vi "EvaluateOpStateExit.vi"(8 "error in (no error)":errorcluster, 9 "data":T2, 10 "config in":T1, 11 "Qbus in":refnum<class "Qbus.lvclass">) -> (0 "error out":errorcluster, 2 "config out":T1, 3 "Qbus out":refnum<class "Qbus.lvclass">)   [LabVIEW 2017, in "McsaDataEventCreator.lvlib"]
uses:
  <vilib>/addons/InsightCM/Devices/Shared/Mcsa/McsaDataEventCreator/McsaDataEventCreator.lvlib
  <vilib>/addons/InsightCM/Devices/Shared/Common/DataFlow/controls/Data.ctl
  <vilib>/addons/InsightCM/Utilities/DataAccessors/controls/wfmSGL_DVR.ctl
  <vilib>/addons/PointValueMap/controls/PointMap.ctl
  <vilib>/addons/InsightCM/Devices/Shared/Common/DataFlow/controls/Type.ctl
  <vilib>/addons/Qbus/Qbus.lvclass
  <vilib>/addons/InsightCM/Devices/Shared/Mcsa/McsaDataEventCreator/controls/config.ctl
  <vilib>/addons/InsightCM/Devices/Shared/Mcsa/McsaDataEventCreator/controls/AcqParams.ctl
  <vilib>/addons/InsightCM/Devices/Shared/Common/DataAccumulator/controls/AccumulationSettings.ctl
  <vilib>/addons/InsightCM/Devices/Shared/Common/DataAccumulator/controls/accumulationType.ctl
  <vilib>/addons/InsightCM/Devices/Shared/Common/DVRBuffer/controls/BufferLocation.ctl
  <vilib>/addons/InsightCM/Devices/Shared/Mcsa/McsaDataEventCreator/controls/DataEventConfig.ctl
  <vilib>/addons/InsightCM/Devices/Shared/Common/DataEventCreator/controls/Reason.ctl
  <vilib>/addons/PointValueMap/subVIs/Point_Read_string.vi
  <vilib>/addons/PointValueMap/PointValueMap.lvlib
  <vilib>/addons/InsightCM/Devices/Shared/Common/DataEventCreator/DataEventCreator.lvlib
  <vilib>/addons/InsightCM/Devices/Shared/Common/DVRBuffer/DVRBuffer.lvlib
  <vilib>/addons/InsightCM/Devices/Shared/Common/DataAccumulator/DataAccumulator.lvlib
  <vilib>/addons/InsightCM/Devices/Shared/Common/DataFlow/DataFlow.lvlib
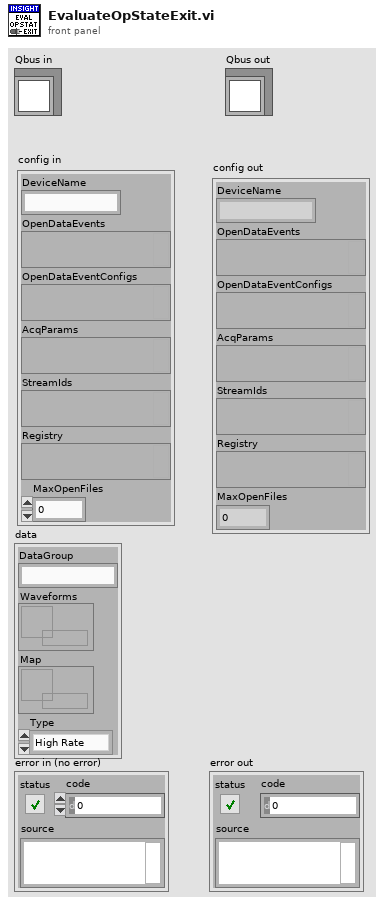
[diagram p1: front panel]
types:
  T1 = typedef "McsaDataEventCreator.lvlib/config.ctl" = cluster{"DeviceName":string, "OpenDataEvents":variant, "OpenDataEventConfigs":variant, "AcqParams":variant, "StreamIds":variant, "Registry":variant, "MaxOpenFiles":i32}
  T2 = typedef "DataFlow.lvlib/Data.ctl" = cluster{"DataGroup":string, "Waveforms":T3, "Map":T4, "Type":T5}
  T3 = typedef "wfmSGL_DVR.ctl" = refnum<data-value>
  T4 = typedef "PointValueMap.lvlib/PointMap.ctl" = refnum<data-value>
  T5 = typedef "DataFlow.lvlib/Type.ctl" = enum16{"High Rate", "Low Rate", "Burst Mode"}
  T6 = typedef "McsaDataEventCreator.lvlib/AcqParams.ctl" = cluster{"Stream":bool, "PreTrigger":i32, "CollectOnEnter":bool, "Enter PreTrigger":i32, "Enter Length":dbl, "CollectOnExit":bool, "ContinuousData":bool, "Accumulation Settings":T7}
  T7 = typedef "DataAccumulator.lvlib/AccumulationSettings.ctl" = cluster{"Type":T8, "Length":dbl, "Max Time (sec)":dbl, "Start Block":T9, "Acquired (sec)":dbl, "Acquired (pulses)":i32, "Initial Pulse Offset":dbl, "Stop Block":T9, "LastBlockAdded":u32}
  T8 = typedef "DataAccumulator.lvlib/accumulationType.ctl" = enum16{"none", "seconds", "revolutions"}
  T9 = typedef "DVRBuffer.lvlib/BufferLocation.ctl" = cluster{"Block":u32, "Index":i32}
  T10 = typedef "DataEventCreator.lvlib/Reason.ctl" = enum16{"Periodic Event", "Delta EU Event", "Trend Event", "Alarm Event", "User Event", "Enter Operating State", "Exit Operating State", "Multiple Events", "Other"}
  T11 = typedef "McsaDataEventCreator.lvlib/DataEventConfig.ctl" = cluster{"AcqParams":T6, "OpState":string, "ExitOpState":bool, "Reason":string, "StreamId":string, "Map":T4, "DataSetIds":variant, "IncludeWaveforms":bool, "TrendPointsOnly":bool}
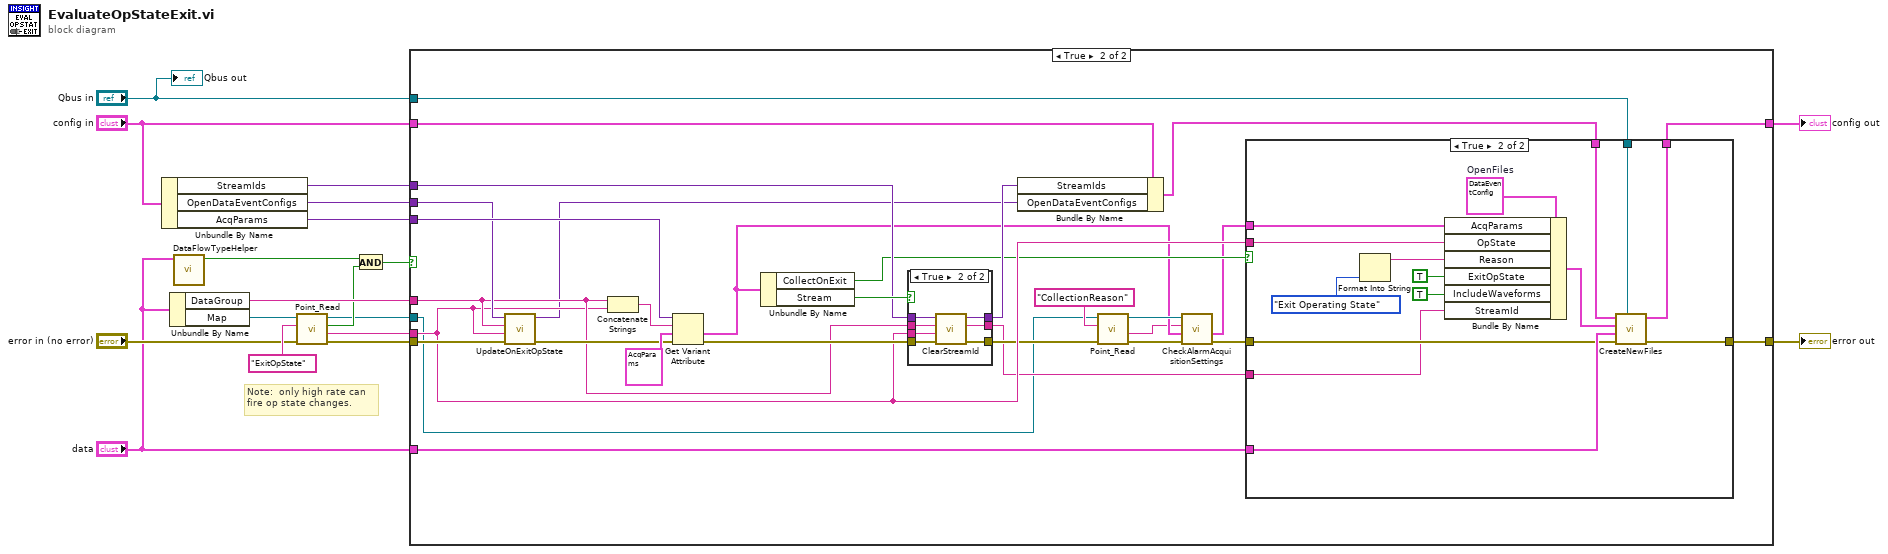
[diagram p0: block diagram]
diagram:
  # "Note:  only high rate can\nfire op state changes."
  n1 = Unbundle By Name("config in") -> ("StreamIds"=w12:variant, "OpenDataEventConfigs"=w8:variant, "AcqParams"=w7:variant)
  n2 = Unbundle By Name("data") -> ("DataGroup"=w13:string, "Map"=w18:T4)
  n3 = call <vilib>:"DataFlowTypeHelper.vi"("data"="data") -> ("high rate"=w1:bool)  [unwired: 8 in, 2 out]
  n4 = call-poly <vilib>:"Point_Read.vi"("Error In"="error in (no error)", "Tag"="ExitOpState", "Map"=w18) -> ("Error Out"=w15:errorcluster, "Value"=w14:string, "Found?"=w5:bool, "Map Out"=w3:T4)  [unwired: 3 in, 2 out]
  n5 = And(x=w1, y=w5) -> (x .and. y?=w4:bool)
  n6 = case shown="True" w4 {
    tunnel: w15 -> [w19 w37]
    tunnel: w14 -> [_ w33]
    tunnel: w13 -> [_ w34]
    tunnel: w7 -> [_ w49]
    tunnel: w12 -> [_ w45]
    tunnel: "config in" -> [w20 w44]
    tunnel: [w20 w43] -> w10
    tunnel: "data" -> [_ w42]
    tunnel: "Qbus in" -> [_ w41]
    tunnel: [w19 w40] -> w9
    tunnel: w8 -> [_ w35]
    tunnel: w3 -> [_ w25]
    frame False {
    }
    frame True {
      n7 = call <vilib>:"UpdateOnExitOpState.vi"("error in (no error)"=w37, "operating state"=w33, "data group"=w34, "open data event configs in"=w35) -> ("error out"=w36:errorcluster, "open data event configs out"=w32:variant)  [unwired: 6 in]
      n8 = Concatenate Strings(w34, w33) -> (w50:string)
      n9 = Get Variant Attribute(Variant=w49, name=w50, default value (empty Variant)=T6 {"Stream"=FALSE, "PreTrigger"=0, "CollectOnEnter"=FALSE, "Enter PreTrigger"=0, "Enter Length"=0.0, "CollectOnExit"=FALSE, "ContinuousData"=FALSE, "Accumulation Settings"={"Type"=enum."none", "Length"=0.0, "Max Time (sec)"=0.0, "Start Block"={"Block"=0, "Index"=0}, "Acquired (sec)"=0.0, "Acquired (pulses)"=0, "Initial Pulse Offset"=0.0, "Stop Block"={"Block"=0, "Index"=0}, "LastBlockAdded"=0}} ("AcqParams"), error in=w36) -> (value=w22:T6, error out=w46:errorcluster)  [unwired: 2 out]
      n10 = Unbundle By Name(w22) -> ("CollectOnExit"=w31:bool, "Stream"=w47:bool)
      n11 = case shown="True" w47 {
        tunnel: w46 -> [w68 w76]
        tunnel: w45 -> [w69 w75]
        tunnel: w34 -> [_ w74]
        tunnel: w33 -> [_ w73]
        tunnel: [w69 w72] -> w39
        tunnel: [_ w71] -> w27
        tunnel: [w68 w70] -> w29
        frame False {
        }
        frame True {
          n12 = call <vilib>:"ClearStreamId.vi"("error in (no error)"=w76, "operating state"=w73, "data group"=w74, "OpStateCorrIds in"=w75) -> ("error out"=w70:errorcluster, "operating state corrId"=w71:string, "OpStateCorrIds out"=w72:variant)  [unwired: 5 in]
        }
      }
      n13 = Bundle By Name(cluster=w44, "StreamIds"=w39, "OpenDataEventConfigs"=w32) -> (w38:T1)
      n14 = call-poly <vilib>:"Point_Read.vi"("Error In"=w29, "Tag"="CollectionReason", "Map"=w25) -> ("Error Out"=w24:errorcluster, "Value"=w21:string, "Map Out"=w26:T4)  [unwired: 3 in, 3 out]
      n15 = call <vilib>:"CheckAlarmAcquisitionSettings.vi"("error in (no error)"=w24, "acq config in"=w22, "collection reason"=w21, "map"=w26) -> ("error out"=w28:errorcluster, "acq config out"=w23:T6)  [unwired: 6 in]
      n16 = case shown="True" w31 {
        tunnel: w23 -> [_ w67]
        tunnel: [w52 w66] -> w43
        tunnel: w42 -> [_ w65]
        tunnel: w41 -> [_ w64]
        tunnel: [w51 w63] -> w40
        tunnel: w28 -> [w51 w62]
        tunnel: w38 -> [w52 w61]
        tunnel: w33 -> [_ w60]
        tunnel: w27 -> [_ w54]
        frame False {
        }
        frame True {
          w59 = T11 {"AcqParams"={"Stream"=FALSE, "PreTrigger"=0, "CollectOnEnter"=FALSE, "Enter PreTrigger"=0, "Enter Length"=0.0, "CollectOnExit"=FALSE, "ContinuousData"=FALSE, "Accumulation Settings"={"Type"=enum."none", "Length"=0.0, "Max Time (sec)"=0.0, "Start Block"={"Block"=0, "Index"=0}, "Acquired (sec)"=0.0, "Acquired (pulses)"=0, "Initial Pulse Offset"=0.0, "Stop Block"={"Block"=0, "Index"=0}, "LastBlockAdded"=0}}, "OpState"="", "ExitOpState"=FALSE, "Reason"="", "StreamId"="", "Map"=refnum, "DataSetIds"=variant, "IncludeWaveforms"=FALSE, "TrendPointsOnly"=FALSE}  # OpenFiles
          n17 = Format Into String(Reason."Exit Operating State" ("Reason")) -> (resulting string=w55:string)  [unwired: 3 in, 1 out]
          n18 = Bundle By Name(cluster=w59, "AcqParams"=w67, "OpState"=w60, "Reason"=w55, "ExitOpState"=TRUE, "IncludeWaveforms"=TRUE, "StreamId"=w54) -> (w58:T11)
          n19 = call <vilib>:"CreateNewFiles.vi"("Qbus"=w64, "error in (no error)"=w62, "data flow"=w65, "data event config"=w58, "config"=w61) -> ("error out"=w63:errorcluster, "config out"=w66:T1)  [unwired: 5 in]
        }
      }
    }
  }
  "error out" <- w9
  "config out" <- w10
  "Qbus out" <- "Qbus in"
